vi "Main.vi"(8 "error in":errorcluster, 9 "Error Queue":refnum<queue>, 10 "Controller Queue":refnum<queue>, 11 "Application Events":refnum<user-event>) -> (0 "error out":errorcluster)   [LabVIEW 2020, in "Sensor Interface.lvlib"]
uses:
  Sensor Interface.lvlib
  Controller/Controls/Module Message.ctl
  Controller/Controls/Application Modules.ctl
  Controller/Controls/Application Event Message.ctl
  Controller/Controls/Application Events.ctl
  Controls/Module Loop Data.ctl
  Controller/Controller.lvlib
panel:
  in  "Elevator Position":i32(slide)=1 min=1 max=4 step=1 scale=1.0..4.0
  # "[Covers: UI4] \n[Covers: UI4A]"
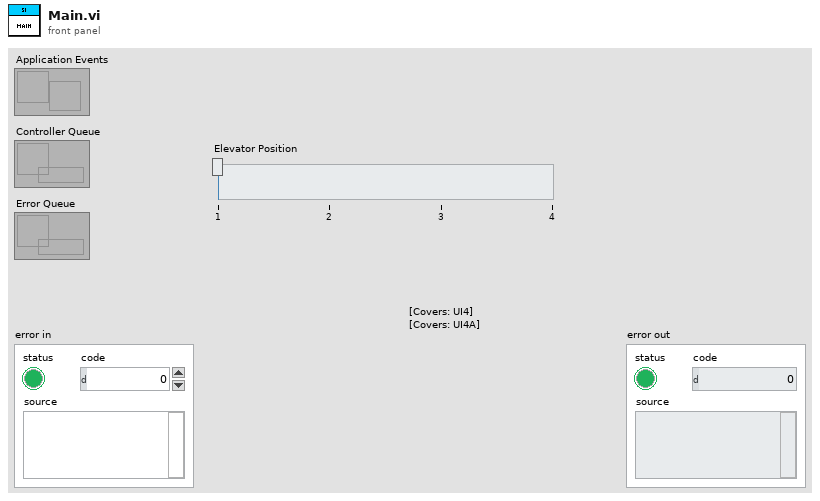
[diagram p1: front panel]
types:
  T1 = typedef "Sensor Interface.lvlib/Module Loop Data.ctl" = cluster{"Timing":cluster{"IsTiming?":bool, "Time Target Sec":dbl, "Time Ticks Ms":i32, "Time Ticks Counter":i32}}
  T2 = typedef "Controller.lvlib/Application Events.ctl" = enum16{"Controller: Initialize", "Controller: Initialize Start And Move State", "Controller: Initialize Analysis State", "Controller: Initialize Continue Travel State", "Controller: Initialize Stop At Floor", "Controller: Initialize Open And Close Door Sequence", "Controller: Initialize No Request Remaining", "Controller: Initialize Emergency Call", "Controller: Initialize Terminate Process", "Controller: Publish State", "UI: Elevator Call", "UI: Broadcast State", "UI: Next Destination Reached", "UI: Timeout Reached", "UI: Emergency Call", "UI: Terminate State", "UI: Door Opened", "UI: Door Closed", "UI: Floor Reached", "UI: Door About To Close"}
  T3 = typedef "Controller.lvlib/Application Event Message.ctl" = cluster{"Source":T4, "Event":T2, "Data":variant}
  T4 = typedef "Controller.lvlib/Application Modules.ctl" = enum16{"Controller", "User Console", "Display Console", "Sensor Interface", "Configuration Database", "Error Module"}
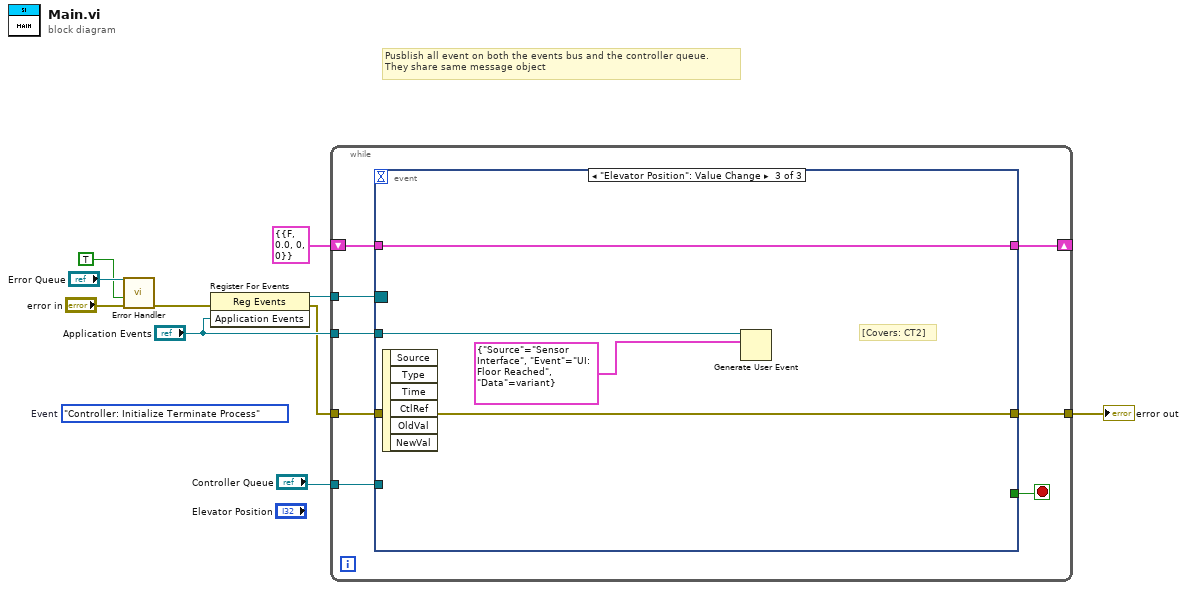
[diagram p0: block diagram]
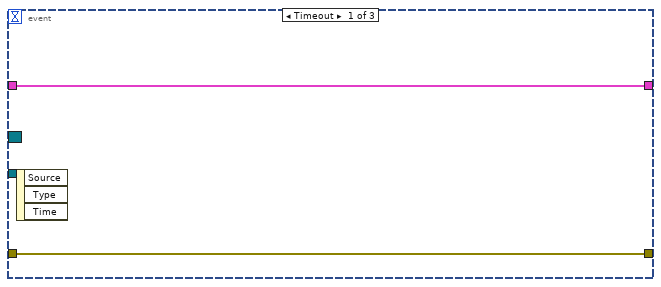
[diagram p2: hidden frame]
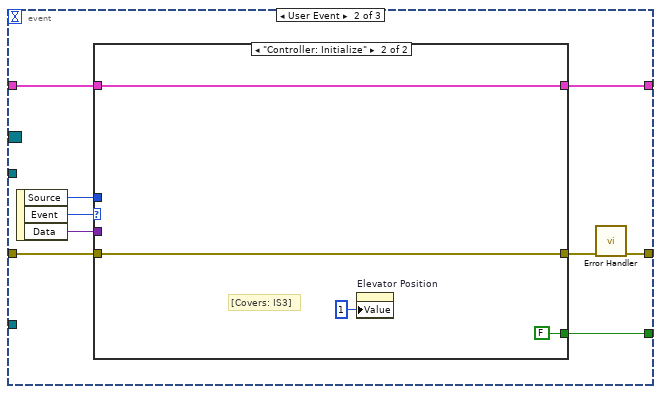
[diagram p3: hidden frame]
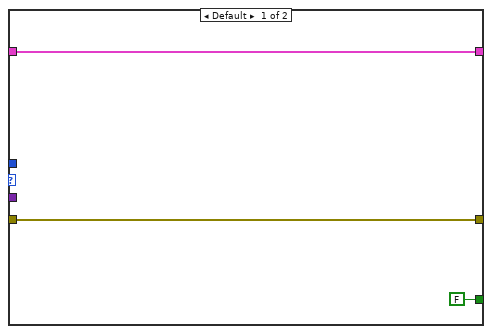
[diagram p4: hidden frame]
diagram:
  (unwired) Application_Events."Controller: Initialize Terminate Process"  # Event
  # "Pusblish all event on both the events bus and the controller queue. \nThey share same message object"
  n1 = call "Error Handler.vi"("error in"="error in", "Load Reference?"=TRUE, "Error Queue"="Error Queue") -> ("error out"=w4:errorcluster)  [unwired: 8 in]
  n2 = register-events(error in=w4, "Application Events") -> (reference out=w9:refnum<event-registration>, error out=w3:errorcluster)  [unwired: 1 in]
  n3 = while {
    tunnel: "Application Events" -> [w18]
    tunnel: w9 -> [w17]
    tunnel: w3 -> [w16]
    tunnel: "Controller Queue" -> [w15]
    tunnel: [w13] -> w2
    shift-right: [w12] -> _
    shift-left: T1 {"Timing"={"IsTiming?"=FALSE, "Time Target Sec"=0.0, "Time Ticks Ms"=0, "Time Ticks Counter"=0}} ("Event Loop Data") -> [w11]
    stop <- w14 stop-if-true
    n4 = event shown="[2] \"Elevator Position\": Value Change" {
      selector: w17 -> [_ _ _]
      dyn-events: _ -> [_ _ _]
      timeout: _ -> [_ _ _]
      tunnel: w18 -> [_ _ w38]
      tunnel: w16 -> [w20 w25 w40]
      tunnel: w15 -> [_ _ _]
      tunnel: [_ w26 _] -> w14
      tunnel: [w20 w23 w40] -> w13
      tunnel: [w19 w22 w39] -> w12
      tunnel: w11 -> [w19 w21 w39]
      event Timeout {
        n5 = event-data() -> ()  [unwired: 1 in, 3 out]
      }
      event User Event {
        n6 = event-data() -> ("Source"=w28:T4, "Event"=w29:T2, "Data"=w27:variant)  [unwired: 1 in]
        n7 = case shown="\"Controller: Initialize\"" w29 {
          tunnel: w28 -> [_ _]
          tunnel: w27 -> [_ _]
          tunnel: [FALSE FALSE] -> w26
          tunnel: [w31 w35] -> w24
          tunnel: w25 -> [w31 w35]
          tunnel: [w30 w33] -> w22
          tunnel: w21 -> [w30 w33]
          frame Default {
          }
          frame "Controller: Initialize" {
            # "[Covers: IS3]"
            n8 = property on="Elevator Position" class="Slide (strict)"("Value"=1 ("Elevator Position")) -> ()  [unwired: 2 in, 2 out]
          }
        }
        n9 = call "Error Handler.vi"("error in"=w24) -> ("error out"=w23:errorcluster)  [unwired: 10 in]
      }
      event "Elevator Position": Value Change {
        # "[Covers: CT2]"
        n10 = event-data() -> ()  [unwired: 1 in, 6 out]
        n11 = Generate User Event(user event=w38, event data cluster=T3 {"Source"=enum."Sensor Interface", "Event"=enum."UI: Floor Reached", "Data"=variant} ("event data")) -> ()  [unwired: 2 in, 2 out]
      }
    }
  }
  "error out" <- w2
